vi "Chronos TDMS Load Channel Table from TDMS Properties.vi"(8 "error in (no error)":errorcluster, 11 "file path":path) -> (0 "error out":errorcluster, 3 "Channels":T1[](array[typedef])=[{"Physical"={"Type"=enum."NI cRIO", "Device"="", "Channel"=0}, "Name"="test ch", "Measurement"="", "Units"="", "Scaling"={"Scaling Type"=enum."None", "Parameters"=[1.0, 2.0, 3.0, 4.0]}, "Limits"={"Low Red"=0.0, "Low Yellow"=0.0, "Hi Yellow"=0.0, "Hi Red"=0.0}, "Digits"=0, "Alarms"=[], "Config"={"type string"=[], "Configuration Str Var"=""}}, {"Physical"={"Type"=enum."NI cRIO", "Device"="", "Channel"=1}, "Name"="2nd channel", "Measurement"="Temperature", "Units"="C", "Scaling"={"Scaling Type"=enum."Polynomial", "Parameters"=[0.0, 1.0]}, "Limits"={"Low Red"=-3.0, "Low Yellow"=0.0, "Hi Yellow"=0.0, "Hi Red"=0.0}, "Digits"=0, "Alarms"=[], "Config"={"type string"=[], "Configuration Str Var"=""}}])   [LabVIEW 2021]
uses:
  typedefs/Chronos cluster Channel.ctl
  typedefs/Chronos cluster Hardware Configuration Physical.ctl
  Subsystem Modules/Chronos enum Device Hardware Type.ctl
  typedefs/Chronos cluster Scaling.ctl
  typedefs/Chronos enum Scaling Type.ctl
  typedefs/Chronos cluster Limits.ctl
  typedefs/Chronos cluster Alarm.ctl
  typedefs/Chronos enum Alarm Action.ctl
  typedefs/Chronos cluster Channel Configuration variant.ctl
panel:
  out "All Errors":errorcluster[](array[cluster])
  in  "Channel":T1
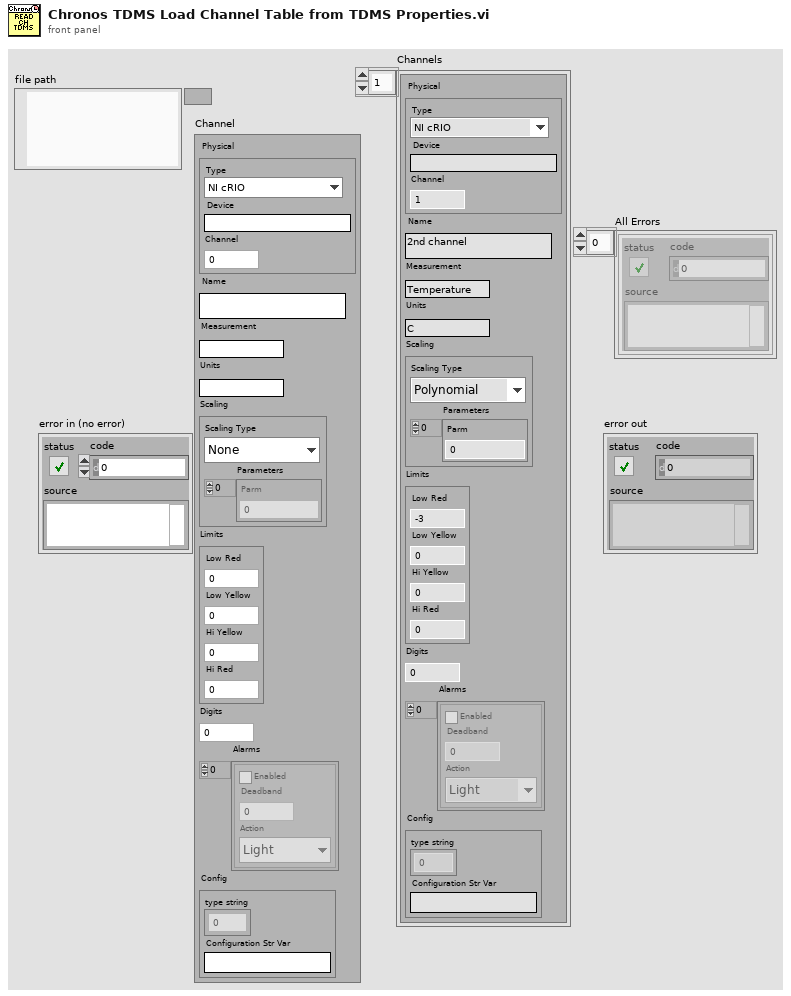
[diagram p1: front panel]
types:
  T1 = typedef "Chronos cluster Channel.ctl" = cluster{"Physical":T2, "Name":string, "Measurement":string, "Units":string, "Scaling":T4, "Limits":T6, "Digits":i32, "Alarms":T7[], "Config":T9}
  T2 = typedef "Chronos cluster Hardware Configuration Physical.ctl" = cluster{"Type":T3, "Device":string, "Channel":i32}
  T3 = typedef "Chronos enum Device Hardware Type.ctl" = enum16{"NI cRIO", "Keithley 3706"}
  T4 = typedef "Chronos cluster Scaling.ctl" = cluster{"Scaling Type":T5, "Parameters":dbl[]}
  T5 = typedef "Chronos enum Scaling Type.ctl" = enum16{"None", "Polynomial"}
  T6 = typedef "Chronos cluster Limits.ctl" = cluster{"Low Red":dbl, "Low Yellow":dbl, "Hi Yellow":dbl, "Hi Red":dbl}
  T7 = typedef "Chronos cluster Alarm.ctl" = cluster{"Enabled":bool, "Deadband":i32, "Action":T8}
  T8 = typedef "Chronos enum Alarm Action.ctl" = enum16{"Light", "Message", "Safe"}
  T9 = typedef "Chronos cluster Channel Configuration variant.ctl" = cluster{"type string":i16[], "Configuration Str Var":string}
  T10 = enum16{"open", "open or create", "create or replace", "create", "open (read-only)"}
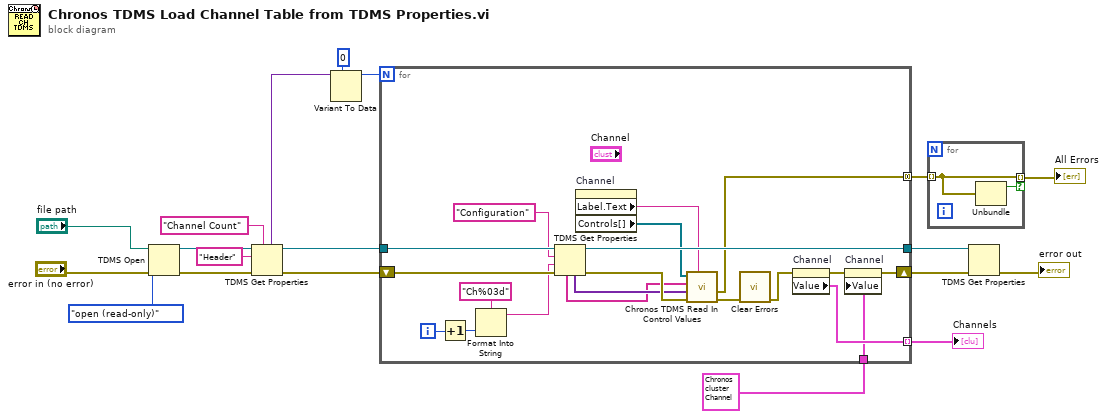
[diagram p0: block diagram]
diagram:
  n1 = TDMS Open(8:"error in (no error)", 10:T10."open (read-only)" ("operation (0:open)"), 11:"file path") -> (0:w18:errorcluster, 3:w17:refnum<k34>)  [unwired: 4 in]
  n2 = TDMS Get Properties(7:"Channel Count" ("property name"), 8:w18, 10:"Header" ("group name"), 11:w17) -> (0:w11:errorcluster, 3:w5:refnum<k34>, 4:w14:variant)  [unwired: 2 in, 3 out]
  n3 = Variant To Data(type=0, Variant=w14) -> (data=w12:i32)  [unwired: 1 in, 1 out]
  n4 = for {
    N: w12 -> [_]
    shift-right: [w23] -> w10
    shift-left: w11 -> [w39]
    tunnel: w5 -> [w38]
    tunnel: [w36] -> w9
    tunnel: [w34] -> w7 mode=indexing
    tunnel: [w29] -> w4 mode=concatenating
    tunnel: T1 {"Physical"={"Type"=enum."NI cRIO", "Device"="", "Channel"=1}, "Name"="2nd channel", "Measurement"="Temperature", "Units"="C", "Scaling"={"Scaling Type"=enum."Polynomial", "Parameters"=[]}, "Limits"={"Low Red"=-3.0, "Low Yellow"=0.0, "Hi Yellow"=0.0, "Hi Red"=0.0}, "Digits"=0, "Alarms"=[], "Config"={"type string"=[], "Configuration Str Var"=""}} ("Channel") -> [w21]
    i -> [w37]
    n5 = Increment(x=w37) -> (x+1=w27:i32)
    n6 = Format Into String(format string="Ch%03d", w27) -> (resulting string=w25:string)  [unwired: 2 in, 1 out]
    n7 = TDMS Get Properties(8:w39, 9:w25, 10:"Configuration", 11:w38) -> (0:w35:errorcluster, 3:w36:refnum<k34>, 4:w33:variant[], 6:w24:string[])  [unwired: 2 in, 2 out]
    n8 = property on="Channel" class="Clust (strict)"() -> ("Label.Text"=w32:string, "Controls[]"=w20:refnum<vi>[])  [unwired: 2 in, 2 out]
    n9 = call "Chronos TDMS Read In Control Values.vi"("Parent"=w32, "error in (no error)"=w35, "Values"=w33, "Properties"=w24, "Controls"=w20) -> ("error out"=w31:errorcluster, "All Errors"=w29:errorcluster[])  [unwired: 5 in]
    n10 = call <vilib>:"Clear Errors.vi"("error in (no error)"=w31) -> ("error out"=w30:errorcluster)  [unwired: 5 in, 1 out]
    n11 = property on="Channel" class="Clust (strict)"(error in=w30) -> (error out=w22:errorcluster, "Value"=w34:T1)  [unwired: 1 in, 1 out]
    n12 = property on="Channel" class="Clust (strict)"(error in=w22, "Value"=w21) -> (error out=w23:errorcluster)  [unwired: 1 in, 1 out]
  }
  "Channels" <- w7
  n13 = for {
    tunnel: w4 -> [w41] mode=indexing
    tunnel: [w41] -> w3 mode=indexing if=w40
    n14 = Unbundle(w41) -> ("status"=w40:bool)  [unwired: 2 out]
  }
  "All Errors" <- w3
  n15 = TDMS Get Properties(8:w10, 11:w9) -> (0:→"error out":errorcluster)  [unwired: 4 in, 5 out]
